vi "Add to Private Data.vi"(6 "Variant in":variant, 7 "Shift Pressed?":bool, 8 "error in (no error)":errorcluster, 10 "QD Combo Box Ref":refnum<vi>, 11 "QD Launch VI Ref":refnum<vi>) -> (0 "error out":errorcluster, 4 "Variant out":variant)   [LabVIEW 2020, in "Add to Private Data.lvlib"]
doc: "This QuickDrop plugin adds the highlighted data terminals to a class's private data cluster. When the shift key is held, this action adds a reference to the terminal, rather than the value itself.\n\nDefault Shortcut - [O]"
uses:
  Add to Private Data.lvlib
panel:
  in  "Undo Name":string="Quick Drop Keyboard Shortcut"
  # "Do not change the connector pane of this VI.\n\nSee the block diagram for directions on how to use this template."
  # "Specify the name of the Undo transaction"
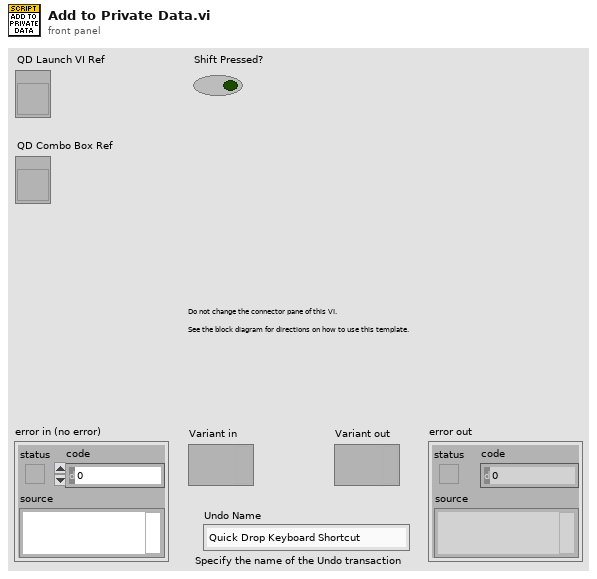
[diagram p1: front panel]
types:
  T1 = typedef "Add to Private Data.lvlib/Private Data Refs.ctl" = cluster{"VI Ref":refnum<vi>, "Panel Ref":refnum<vi>, "Cluster Ref":refnum<vi>}
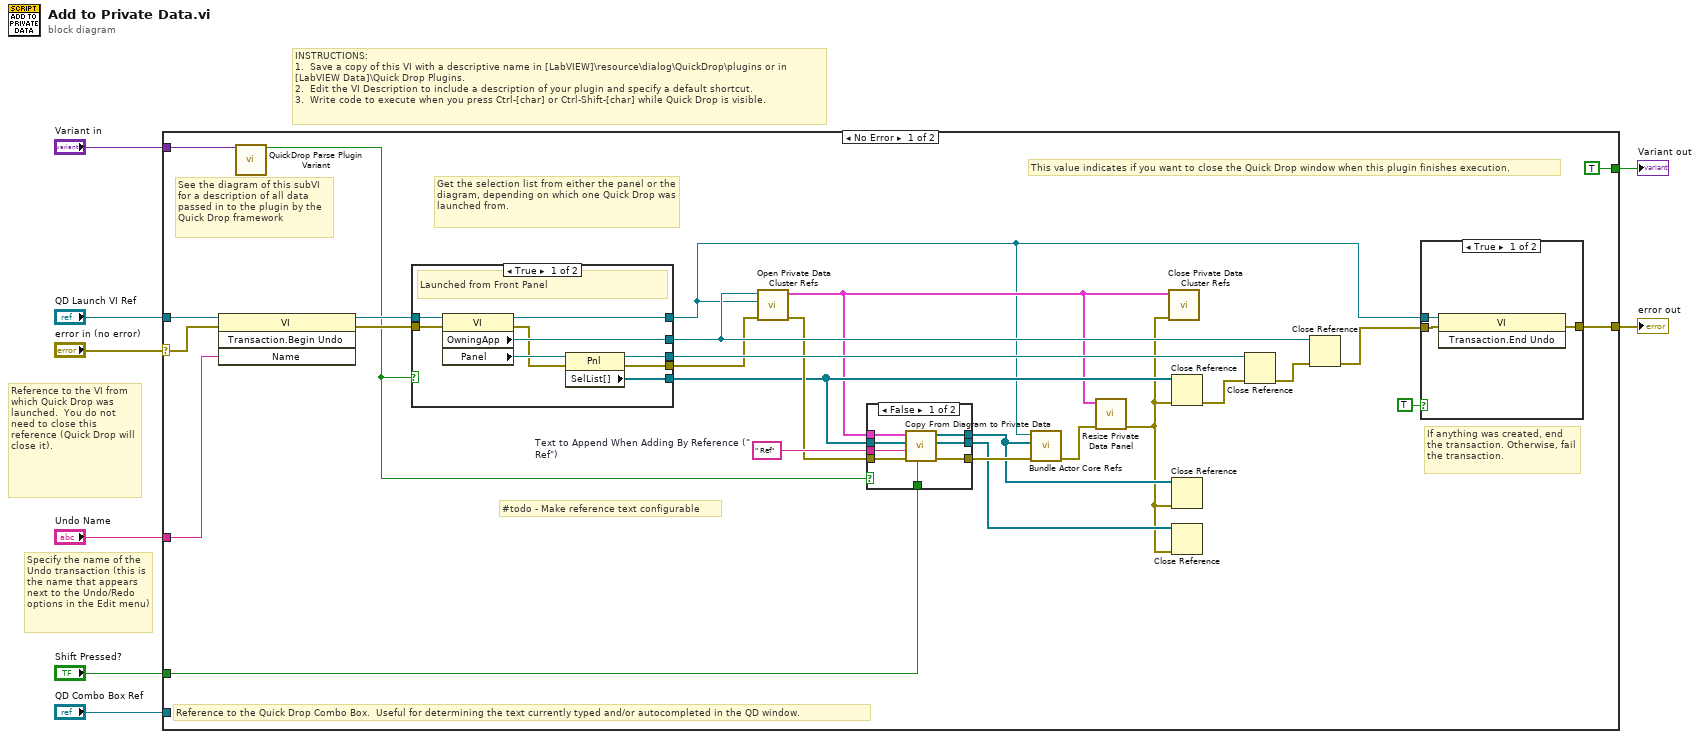
[diagram p0: block diagram]
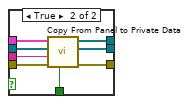
[diagram p2: hidden frame]
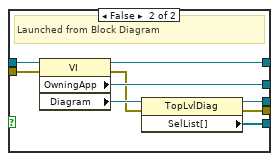
[diagram p3: hidden frame]
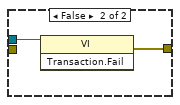
[diagram p4: hidden frame]
diagram:
  # "Specify the name of the Undo transaction (this is the name that appears next to the Undo/Redo options in the Edit menu)"
  # "Reference to the VI from which Quick Drop was launched.  You do not need to close this reference (Quick Drop will close it)."
  # "INSTRUCTIONS:\n1.  Save a copy of this VI with a descriptive name in [LabVIEW]\\resource\\dialog\\QuickDrop\\plugins or in [LabVIEW Data]\\Quick Drop Plugins.\n2.  Edit the VI Description to include a description of your plugin and specify a default shortcut. \n3.  Write code to execute when you press Ctrl-[char] or Ctrl-Shift-[char] while Quick Drop is visible."
  n1 = case shown="No Error" "error in (no error)" {
    selector: "error in (no error)" -> [w35 w75]
    tunnel: [w30 w75] -> w1
    tunnel: "QD Launch VI Ref" -> [w34 _]
    tunnel: "Shift Pressed?" -> [w25 _]
    tunnel: "QD Combo Box Ref" -> [_ _]
    tunnel: "Variant in" -> [w26 _]
    tunnel: "Undo Name" -> [w33 _]
    tunnel: [TRUE _] -> w2
    frame No Error {
      w24 = " Ref"  # Text to Append When Adding By Reference (" Ref")
      # "#todo - Make reference text configurable"
      # "See the diagram of this subVI for a description of all data passed in to the plugin by the Quick Drop framework"
      # "Get the selection list from either the panel or the diagram, depending on which one Quick Drop was launched from."
      # "If anything was created, end the transaction. Otherwise, fail the transaction."
      # "This value indicates if you want to close the Quick Drop window when this plugin finishes execution."
      # "Reference to the Quick Drop Combo Box.  Useful for determining the text currently typed and/or autocompleted in the QD window."
      n2 = invoke class="VI" method="Transaction.Begin Undo"(reference=w34, error in=w35, "Name"=w33) -> (reference out=w29:refnum<vi>, error out=w31:errorcluster)  [unwired: 1 in, 2 out]
      n3 = call <vilib>:"QuickDrop Parse Plugin Variant.vi"("QDKS Variant in"=w26) -> ("QD Launch VI Panel?"=w12:bool)  [unwired: 12 in, 2 out]
      n4 = case shown="True" w12 {
        tunnel: w31 -> [w60 w69]
        tunnel: w29 -> [w59 w68]
        tunnel: [w57 w66] -> w23
        tunnel: [w56 w65] -> w22
        tunnel: [w54 w63] -> w21
        tunnel: [w53 w62] -> w17
        tunnel: [w52 w61] -> w13
        frame True {
          # "Launched from Front Panel"
          n5 = property class="VI"(reference=w59, error in=w60) -> (reference out=w52:refnum<vi>, error out=w55:errorcluster, "OwningApp"=w56:refnum<vi>, "Panel"=w58:refnum<vi>)
          n6 = property class="Pnl"(reference=w58, error in=w55) -> (reference out=w57:refnum<vi>, error out=w54:errorcluster, "SelList[]"=w53:refnum<vi>[])
        }
        frame False {
          # "Launched from Block Diagram"
          n7 = property class="VI"(reference=w68, error in=w69) -> (reference out=w61:refnum<vi>, error out=w64:errorcluster, "OwningApp"=w65:refnum<vi>, "Diagram"=w67:refnum<vi>)
          n8 = property class="TopLvlDiag"(reference=w67, error in=w64) -> (reference out=w66:refnum<vi>, error out=w63:errorcluster, "SelList[]"=w62:refnum<vi>[])
        }
      }
      n9 = call "Open Private Data Cluster Refs.vi"("error in (no error)"=w21, "Calling VI Ref"=w13, "Application Ref"=w22) -> ("error out"=w19:errorcluster, "Private Data Refs"=w16:T1)  [unwired: 7 in]
      n10 = case shown="False" w12 {
        tunnel: w25 -> [w43 w45]
        tunnel: w24 -> [w42 w49]
        tunnel: w19 -> [w41 w48]
        tunnel: w17 -> [w40 w50]
        tunnel: w16 -> [w39 w51]
        tunnel: [w38 w46] -> w11
        tunnel: [w37 w47] -> w15
        tunnel: [w36 w44] -> w10
        frame False {
          n11 = call "Copy From Diagram to Private Data.vi"("Add as Reference?"=w43, "error in (no error)"=w41, "Text to Append (\" Ref\")"=w42, "GObjects in"=w40, "Private Data Refs"=w39) -> ("error out"=w37:errorcluster, "Other GObjects"=w36:refnum<vi>[], "ControlReferenceConstants"=w38:refnum<vi>[])  [unwired: 4 in]
        }
        frame True {
          n12 = call "Copy From Panel to Private Data.vi"("Add as Reference?"=w45, "error in (no error)"=w48, "Text to Append (\" Ref\")"=w49, "GObjects in"=w50, "Private Data Refs"=w51) -> ("error out"=w47:errorcluster, "Other GObjects"=w44:refnum<vi>[], "ControlReferenceConstants"=w46:refnum<vi>[])  [unwired: 4 in]
        }
      }
      n13 = call "Bundle Actor Core Refs.vi"("error in (no error)"=w15, "ControlReferenceConstants"=w11, "VI"=w13) -> ("error out"=w14:errorcluster)  [unwired: 8 in]
      n14 = call "Resize Private Data Panel.vi"("error in (no error)"=w14, "Private Data Refs"=w16) -> ("error out"=w9:errorcluster)  [unwired: 9 in]
      n15 = call "Close Private Data Cluster Refs.vi"("error in (no error)"=w9, "Private Data Refs"=w16) -> ()  [unwired: 9 in, 1 out]
      n16 = Close Reference(reference=w17, error in (no error)=w9) -> (error out=w18:errorcluster)
      n17 = Close Reference(reference=w11, error in (no error)=w9) -> ()  [unwired: 1 out]
      n18 = Close Reference(reference=w10, error in (no error)=w9) -> ()  [unwired: 1 out]
      n19 = Close Reference(reference=w23, error in (no error)=w18) -> (error out=w20:errorcluster)
      n20 = Close Reference(reference=w22, error in (no error)=w20) -> (error out=w28:errorcluster)
      n21 = case shown="True" TRUE {
        tunnel: w13 -> [w71 w73]
        tunnel: [w72 w74] -> w30
        tunnel: w28 -> [w70 _]
        frame True {
          n22 = invoke class="VI" method="Transaction.End Undo"(reference=w71, error in=w70) -> (error out=w72:errorcluster)  [unwired: 1 in, 2 out]
        }
        frame False {
          n23 = invoke class="VI" method="Transaction.Fail"(reference=w73) -> (error out=w74:errorcluster)  [unwired: 2 in, 2 out]
        }
      }
    }
    frame Error {
    }
  }
  "error out" <- w1
  "Variant out" <- w2
